vi "模块启用.vi"(4 "error in (no error)":errorcluster caption="错误输入（无错误）", 5 "Value":T2 caption="值", 6 "Container State":T3 caption="容器状态", 7 "Display State In":T1={"模块启用"={"环境动力"=FALSE, "氨氮"=FALSE, "总磷"=FALSE, "总氮"=FALSE, "高锰酸盐指数"=FALSE, "化学需氧量"=FALSE, "多参数"=FALSE, "加标回收"=FALSE, "气象"=FALSE, "EXO2"=FALSE, "剖面系统"=FALSE}, "模块名称"={"采配水"="环境动力", "氨氮"="氨氮", "总磷"="总磷", "总氮"="总氮", "高锰酸盐指数"="高锰酸盐指数", "化学需氧量"="化学需氧量", "多参数"="多参数", "加标回收"="加标回收", "气象"="GPS", "EXO2"="EXO2", "剖面系统"="剖面系统"}} caption="显示状态输入") -> (0 "error out":errorcluster caption="错误输出", 3 "Display State Out":T1={"模块启用"={"环境动力"=FALSE, "氨氮"=FALSE, "总磷"=FALSE, "总氮"=FALSE, "高锰酸盐指数"=FALSE, "化学需氧量"=FALSE, "多参数"=FALSE, "加标回收"=FALSE, "气象"=FALSE, "EXO2"=FALSE, "剖面系统"=FALSE}, "模块名称"={"采配水"="环境动力", "氨氮"="氨氮", "总磷"="总磷", "总氮"="总氮", "高锰酸盐指数"="高锰酸盐指数", "化学需氧量"="化学需氧量", "多参数"="多参数", "加标回收"="加标回收", "气象"="GPS", "EXO2"="EXO2", "剖面系统"="剖面系统"}} caption="显示状态输出")   [LabVIEW 2016, in "运维调试菜单.xctl"]
uses:
  <vilib>/_xctls/Container State.ctl
  <vilib>/_xctls/XControlSupport.lvlib
panel:
  # "将以下值显示控件替换为所需类型的显示控件。\n不要从连线板中删除该显示控件或其它显示控件。\n不要更改连线板模式。\n值显示控件应始终位于连线板输出端自顶部起第三个接线端。"
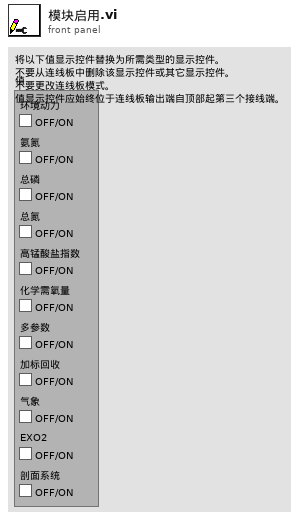
[diagram p1: front panel]
types:
  T1 = typedef "运维调试菜单.xctl/状态 1.ctl" = cluster{"模块启用":T2, "模块名称":cluster{"采配水":string, "氨氮":string, "总磷":string, "总氮":string, "高锰酸盐指数":string, "化学需氧量":string, "多参数":string, "加标回收":string, "气象":string, "EXO2":string, "剖面系统":string}}
  T2 = typedef "运维调试菜单.xctl/模块启用.ctl" = cluster{"环境动力":bool, "氨氮":bool, "总磷":bool, "总氮":bool, "高锰酸盐指数":bool, "化学需氧量":bool, "多参数":bool, "加标回收":bool, "气象":bool, "EXO2":bool, "剖面系统":bool}
  T3 = typedef "XControlSupport.lvlib/Container State.ctl" = cluster{"Indicator?":bool, "Run Mode?":bool, " Refnum":refnum<vi>}
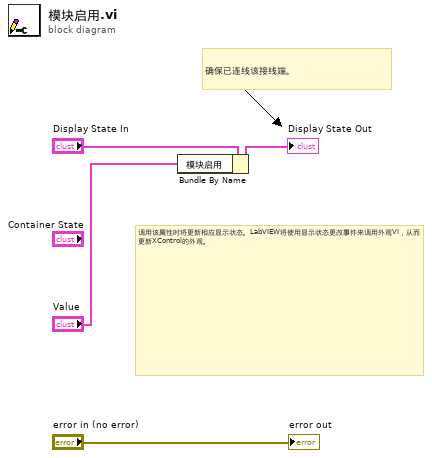
[diagram p0: block diagram]
diagram:
  # "确保已连线该接线端。"
  # "调用该属性时将更新相应显示状态。LabVIEW将使用显示状态更改事件来调用外观VI，从而更新XControl的外观。"
  n1 = Bundle By Name(cluster="Display State In", "模块启用"="Value") -> (→"Display State Out":T1)
  "error out" <- "error in (no error)"
